vi "RF_SetIQCaptureParam.vi"(5 "Param":T1, 7 "RFIndex":u32, 8 "Error In":errorcluster) -> (0 "Error Out":errorcluster, 3 "return":i32)   [LabVIEW 2018]
uses:
  Common/Driver/rd.dll
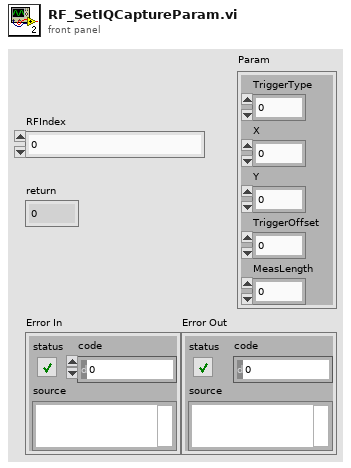
[diagram p1: front panel]
types:
  T1 = cluster{"TriggerType":dbl, "X":dbl, "Y":dbl, "TriggerOffset":dbl, "MeasLength":dbl}
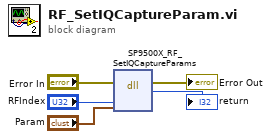
[diagram p0: block diagram]
diagram:
  n1 = dll-call lib="C:/rd/LabVIEW/Common/Driver/rd.dll" fn="SP9500X_RF_SetIQCaptureParams"(error in="Error In", "RFIndex"="RFIndex", "Param"="Param") -> (error out=→"Error Out":errorcluster, "return"=→"return":i32)  [unwired: 4 in, 1 out]
